vi "TestInfo.vi"(7 "Set (f)":bool, 11 "TestInfo 2":T1) -> (3 "TestInfo":T1)   [LabVIEW 2014, in "AnalysisModule.lvlib"]
uses:
  AnalysisModule.lvlib
  TestInfo.ctl
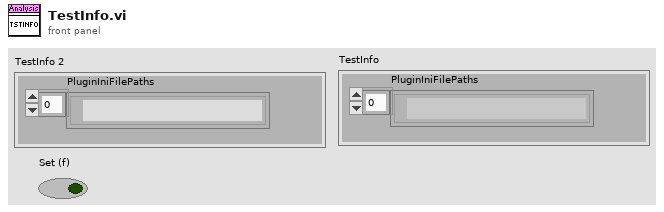
[diagram p1: front panel]
types:
  T1 = typedef "AnalysisModule.lvlib/TestInfo.ctl" = cluster{"PluginIniFilePaths":path[]}
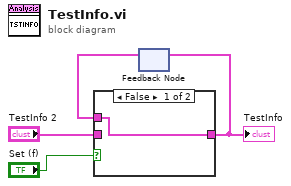
[diagram p0: block diagram]
diagram:
  n1 = feedback #1() -> (w1:T1)  [unwired: 1 in]
  n2 = case shown="False" "Set (f)" {
    tunnel: "TestInfo 2" -> [_ w6]
    tunnel: [w5 w6] -> w2
    tunnel: w1 -> [w5 _]
    frame False {
    }
    frame True {
    }
  }
  "TestInfo" <- w2
  n3 = feedback-in #1(w2) -> ()
